vi "create prop nodes.vi"() -> ()   [LabVIEW 2023]
uses:
  <resource>/Framework/Providers/LVClassLibrary/NewAccessors/MemberVICreation.lvlib
panel:
  out "error out":errorcluster
  in  "Path":path=path "C:/tmp/fix dll import/generation experiment 1/somelib.lvlib"
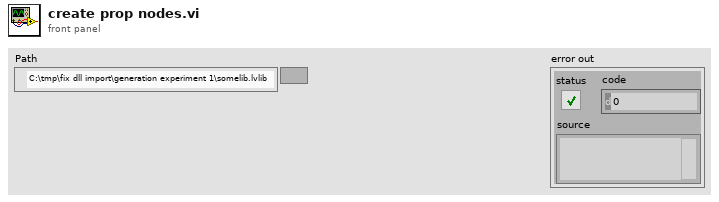
[diagram p1: front panel]
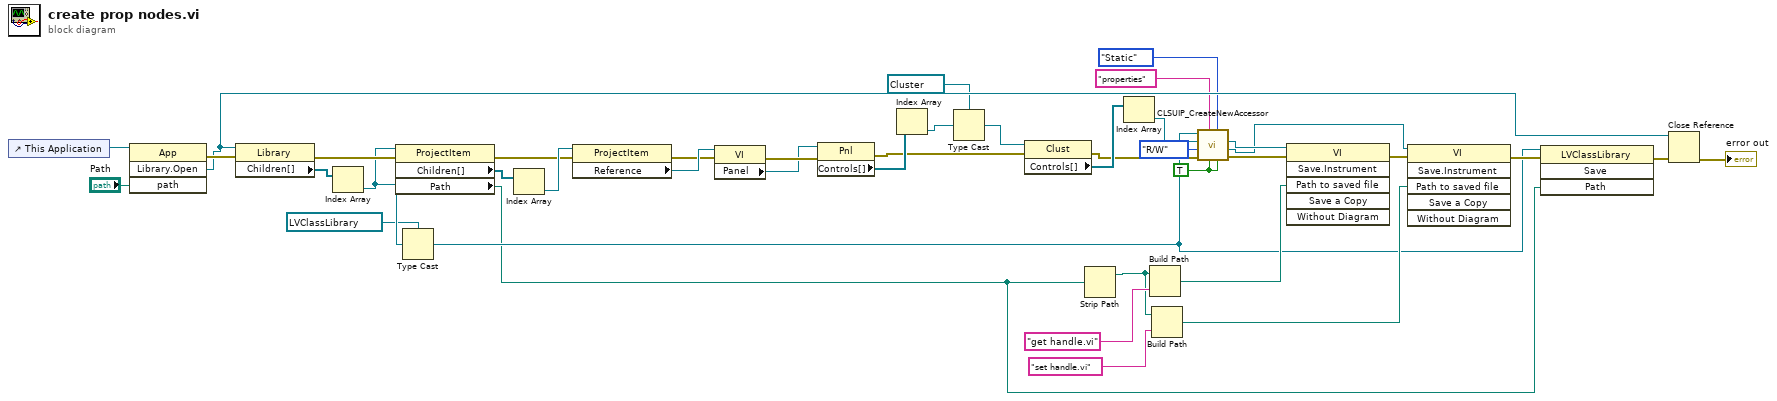
[diagram p0: block diagram]
diagram:
  w18 = TRUE ("Include error terminals")
  n1 = control-ref of="This Application"() -> (w41:refnum<vi>)
  n2 = invoke class="App" method="Library.Open"(reference=w41, "path"="Path") -> (error out=w39:errorcluster, "Open Library"=w36:refnum<vi>)  [unwired: 2 in, 2 out]
  n3 = property class="Library"(reference=w36, error in=w39) -> (error out=w35:errorcluster, "Children[]"=w38:refnum<vi>[])  [unwired: 1 out]
  n4 = Index Array(array=w38) -> (element=w25:refnum<vi>)  [unwired: 1 in]
  n5 = property class="ProjectItem"(reference=w25, error in=w35) -> (error out=w23:errorcluster, "Children[]"=w37:refnum<vi>[], "Path"=w2:path)  [unwired: 1 out]
  n6 = Type Cast(type=refnum<vi> refnum ("element"), x=w25) -> (*(type *) &x=w3:refnum<vi>)
  n7 = Index Array(array=w37) -> (element=w34:refnum<vi>)  [unwired: 1 in]
  n8 = property class="ProjectItem"(reference=w34, error in=w23) -> (error out=w22:errorcluster, "Reference"=w33:refnum<vi>)  [unwired: 1 out]
  n9 = property class="VI"(reference=w33, error in=w22) -> (error out=w32:errorcluster, "Panel"=w31:refnum<vi>)  [unwired: 1 out]
  n10 = property class="Pnl"(reference=w31, error in=w32) -> (error out=w21:errorcluster, "Controls[]"=w30:refnum<vi>[])  [unwired: 1 out]
  n11 = Index Array(array=w30) -> (element=w29:refnum<vi>)  [unwired: 1 in]
  n12 = Type Cast(type=refnum<vi> refnum ("element"), x=w29) -> (*(type *) &x=w27:refnum<vi>)
  n13 = property class="Clust"(reference=w27, error in=w21) -> (error out=w20:errorcluster, "Controls[]"=w26:refnum<vi>[])  [unwired: 1 out]
  n14 = Strip Path(path=w2) -> (stripped path=w11:path)  [unwired: 1 out]
  n15 = Index Array(array=w26) -> (element=w19:refnum<vi>)  [unwired: 1 in]
  n16 = Build Path(base path=w11, name or relative path="get handle.vi" ("Virtual Folder Name")) -> (appended path=w8:path)
  n17 = Build Path(base path=w11, name or relative path="set handle.vi" ("Virtual Folder Name")) -> (appended path=w5:path)
  n18 = call <resource>:"CLSUIP_CreateNewAccessor.vi"("Make available through Property Nodes"=w18, "VI Type"=enum32{"Dynamic", "Static"}."Static", "Include error terminals"=w18, "Virtual Folder Name"="properties", "error in (no error)"=w20, "Access UI"=enum16{"Read", "Write", "R/W"}."R/W", "PDC Item Refnum"=w19, "LVClassLibrary Ref"=w3) -> ("error out"=w9:errorcluster, "Write VI"=w6:refnum<vi>, "Read VI"=w10:refnum<vi>)  [unwired: 1 in]
  n19 = invoke class="VI" method="Save.Instrument"(reference=w10, error in=w9, "Path to saved file"=w8) -> (error out=w7:errorcluster)  [unwired: 3 in, 5 out]
  n20 = invoke class="VI" method="Save.Instrument"(reference=w6, error in=w7, "Path to saved file"=w5) -> (error out=w4:errorcluster)  [unwired: 3 in, 5 out]
  n21 = invoke class="LVClassLibrary" method="Save"(reference=w3, error in=w4, "Path"=w2) -> (error out=w1:errorcluster)  [unwired: 1 in, 3 out]
  n22 = Close Reference(reference=w36, error in (no error)=w1) -> (error out=→"error out":errorcluster)
